vi "UpdateWorld.vi"(8 "error in (no error)":errorcluster, 10 "World in":refnum<class "3D Object.lvclass">, 11 "Control Window in":refnum<class "Control Window.lvclass">) -> (0 "error out":errorcluster, 3 "Control Window out":refnum<class "Control Window.lvclass">)   [LabVIEW 2015, in "Control Window.lvclass"]
uses:
  Control Window.lvclass
  3D Object/3D Object.lvclass
  3D Object/3D Object.lvclass/3D Object.ctl
  Control Window.lvclass/Control Window.ctl
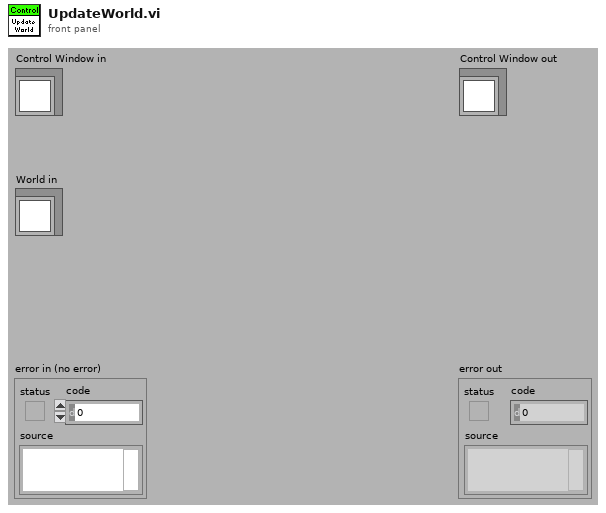
[diagram p1: front panel]
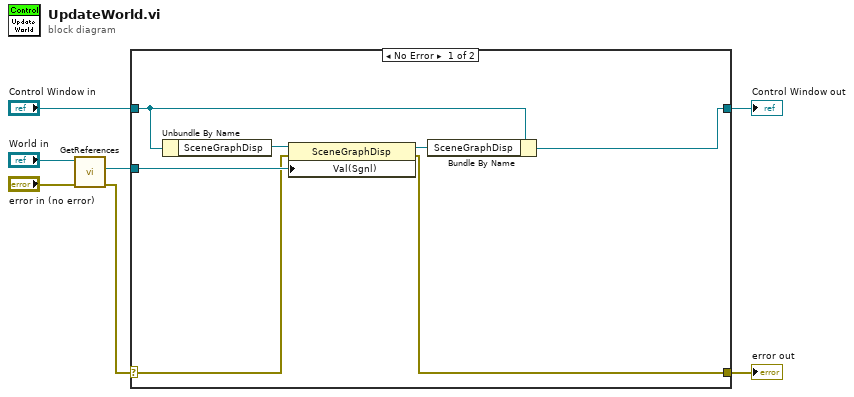
[diagram p0: block diagram]
diagram:
  n1 = call "GetReferences.vi"("error in (no error)"="error in (no error)", "3D Object in"="World in") -> ("error out"=w2:errorcluster, "SceneObject"=w3:refnum<vi>)  [unwired: 6 in, 2 out]
  n2 = case shown="No Error" w2 {
    selector: w2 -> [w9 w16]
    tunnel: [w10 w16] -> w7
    tunnel: [w11 w15] -> w5
    tunnel: "Control Window in" -> [w13 w15]
    tunnel: w3 -> [w14 _]
    frame No Error {
      n3 = Unbundle By Name(w13) -> ("SceneGraphDisp"=w8:refnum<vi>)
      n4 = property class="SceneGraphDisp"(reference=w8, error in=w9, "Val(Sgnl)"=w14) -> (reference out=w12:refnum<vi>, error out=w10:errorcluster)
      n5 = Bundle By Name(cluster=w13, "SceneGraphDisp"=w12) -> (w11:refnum<class "Control Window.lvclass">)
    }
    frame Error {
    }
  }
  "error out" <- w7
  "Control Window out" <- w5
